vi "Rec Destroy - Connection.vi"(8 "error in (no error)":errorcluster, 11 "recordset reference":T2) -> (0 "error out":errorcluster, 3 "connection reference":T1)   [LabVIEW 2017, in "NI_Database_API.lvlib"]
doc: "Frees an object by destroying its associated reference and returns a different reference object. Wire data to the reference input to determine the polymorphic instance to use or manually select the instance."
uses:
  <vilib>/addons/database/NI_Database_API.lvlib
  <vilib>/addons/database/Recordset.llb/Rec ObjectReference.ctl
  <vilib>/addons/database/Connection.llb/Conn ObjectReference.ctl
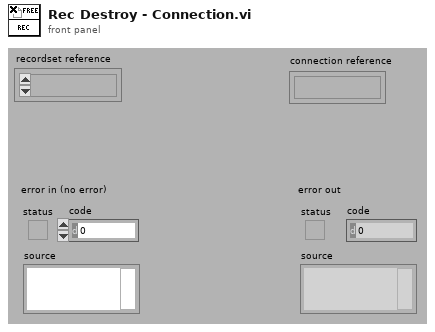
[diagram p1: front panel]
types:
  T1 = typedef "NI_Database_API.lvlib/Conn ObjectReference.ctl" = refnum<k1>
  T2 = typedef "NI_Database_API.lvlib/Rec ObjectReference.ctl" = refnum<k1>
  T3 = typedef "NI_Database_API.lvlib/Rec DataMembers.ctl" = cluster{"ADODB._Recordset":refnum<k7>, "Connection":T1}
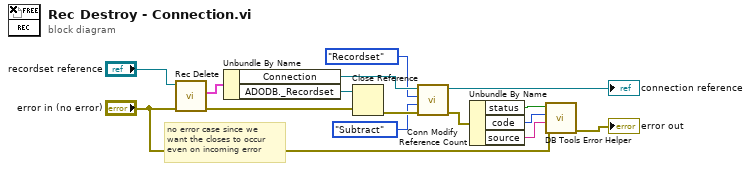
[diagram p0: block diagram]
diagram:
  # "no error case since we\nwant the closes to occur\neven on incoming error"
  n1 = call <vilib>:"Rec Delete.vi"("error in (no error)"="error in (no error)", "recordset reference"="recordset reference") -> ("error out"=w10:errorcluster, "data"=w12:T3)  [unwired: 4 out]
  n2 = Unbundle By Name(w12) -> ("Connection"=w9:T1, "ADODB._Recordset"=w11:refnum<k7>)
  n3 = Close Reference(reference=w11, error in (no error)=w10) -> (error out=w8:errorcluster)
  n4 = call <vilib>:"Conn Modify Reference Count.vi"("error in (no error)"=w8, "operation"=enum16{"Add", "Subtract"}."Subtract" ("Operation"), "object"=enum16{"Recordset", "Command"}."Recordset" ("Object"), "connection reference"=w9) -> ("error out"=w3:errorcluster, "connection reference out"=→"connection reference":T1)  [unwired: 4 out]
  n5 = Unbundle By Name(w3) -> ("status"=w5:bool, "code"=w4:i32, "source"=w2:string)
  n6 = call <vilib>:"DB Tools Error Helper.vi"("Overriding error or warning"="error in (no error)", "source"=w2, "code"=w4, "status"=w5) -> ("error out"=→"error out":errorcluster)  [unwired: 7 out]
